vi "空场混响室吸声量A1计算.vi"(9 "频率":dbl[](array[numeric]), 10 "平均混响时间T1":dbl[](array[numeric])) -> (1 "分立吸声体个数，n":dbl, 2 "混响室吸声量A1":dbl[](array[numeric]))   [LabVIEW 2020]
uses:
  setup/support/rev_setup.lvlib
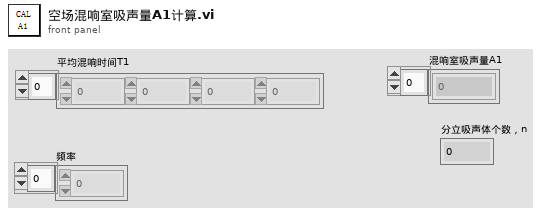
[diagram p1: front panel]
types:
  T1 = typedef "rev_setup.lvlib/EMdata.ctl" = cluster{"大气压力(kPa)":dbl, "大气压力(kPa) 2":dbl, "相对湿度(%)":dbl, "相对湿度(%)2":dbl, "大气温度(℃)":dbl, "大气温度(℃)2":dbl, "声速(m/s)":dbl, "声速(kPa)2":dbl, "混响室容积(立方米) ":dbl, "试件面积(平方米)，S":dbl, "分立吸声体个数，n":dbl}
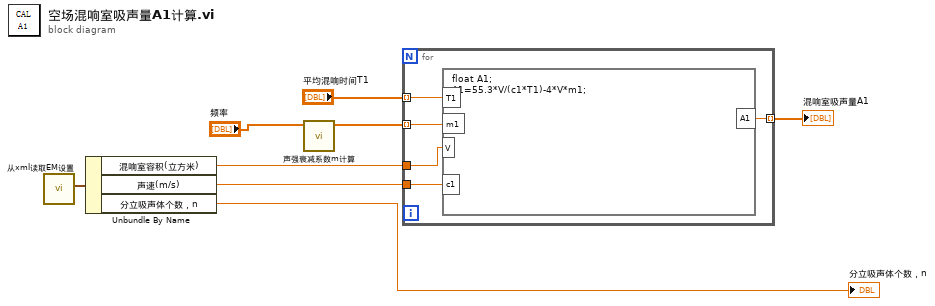
[diagram p0: block diagram]
diagram:
  n1 = call "从xml读取EM设置.vi"() -> ("EM data"=w6:T1)  [unwired: 11 in]
  n2 = Unbundle By Name(w6) -> ("混响室容积(立方米)"=w5:dbl, "声速(m/s)"=w4:dbl, "分立吸声体个数，n"=→"分立吸声体个数，n":dbl)
  n3 = call "声强衰减系数m计算.vi"("输入频率"="频率") -> ("声强衰减系数m1"=w1:dbl[])  [unwired: 9 in, 1 out]
  n4 = for {
    tunnel: "平均混响时间T1" -> [w13] mode=indexing
    tunnel: w5 -> [w12]
    tunnel: w4 -> [w11]
    tunnel: [w10] -> w7 mode=indexing
    tunnel: w1 -> [w9] mode=indexing
    n5 = formula code="float A1;\nA1=55.3*V/(c1*T1)-4*V*m1;"("T1"=w13, "V"=w12, "c1"=w11, "m1"=w9) -> ("A1"=w10:dbl)
  }
  "混响室吸声量A1" <- w7
